vi "resistor2temper.vi"(1 "热敏电阻阻值":dbl) -> (0 "温度":dbl)   [LabVIEW 2015]
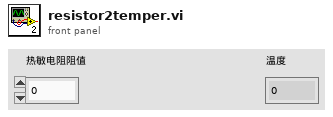
[diagram p1: front panel]
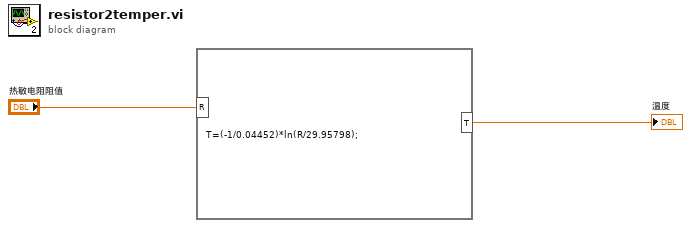
[diagram p0: block diagram]
diagram:
  n1 = formula code="T=(-1/0.04452)*ln(R/29.95798);"("R"="热敏电阻阻值") -> ("T"=→"温度":dbl)
